vi "Update Channel Value.vi"(8 "error in (no error)":errorcluster, 9 "New Value":dbl, 10 "Channel Index":i32, 11 "Output Process in":refnum<class "Random Process.lvclass">) -> (0 "error out":errorcluster, 1 "# elements":u32, 2 "timed out?":bool, 3 "Output Process out":refnum<class "Random Process.lvclass">)   [LabVIEW 2019, in "TimingDRV Engine.lvlib" / "Random Process.lvclass"]
uses:
  Random Process.lvclass
  C:/Users/XEnderMD/Desktop/CD Project Tools/Source/Engine/Parent Classes/Process/Process.lvclass
  Random Process.lvclass/Random Process.ctl
  Parent Classes/Process/Process.lvclass/Process.ctl
  Parent Classes/Process/Process.lvclass
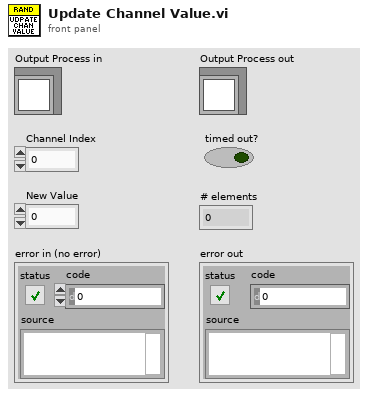
[diagram p1: front panel]
types:
  T1 = typedef "TimingDRV Engine.lvlib/Process.lvclass/Async Paramters.ctl" = cluster{"Device Reference":T2, "Device Clock":string, "Device Inputs FIFO":refnum<k33>, "Device Outputs FIFO":refnum<k33>, "CD Engine Event Ref":T3}
  T2 = typedef "Custom Device API.lvlib/Custom Device Item Ref.ctl" = u64
  T3 = typedef "Custom Device API.lvlib/Custom Device Engine Event Ref.ctl" = refnum<event-registration>
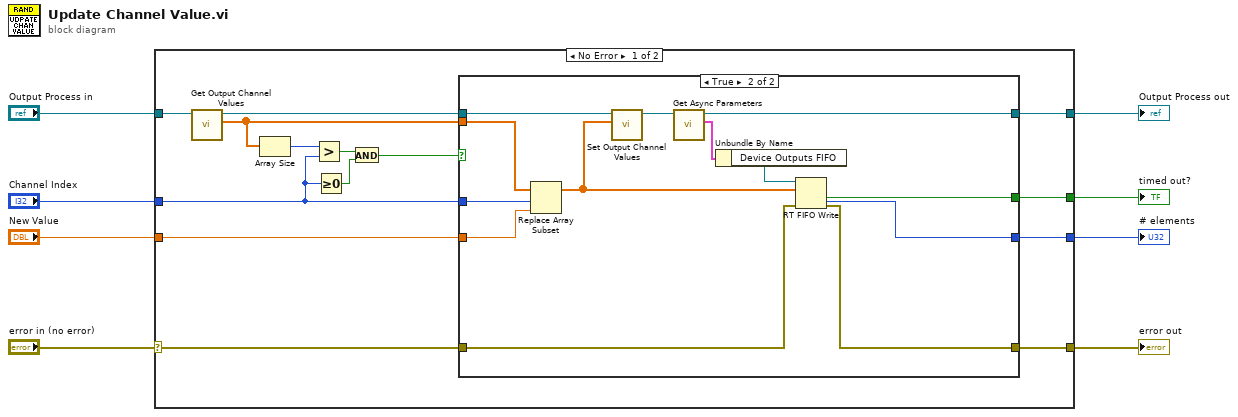
[diagram p0: block diagram]
diagram:
  n1 = case shown="No Error" "error in (no error)" {
    selector: "error in (no error)" -> [w15 w39]
    tunnel: [w22 w38] -> w8
    tunnel: [w21 _] -> w7
    tunnel: [w20 _] -> w6
    tunnel: [w19 w39] -> w5
    tunnel: "New Value" -> [w17 _]
    tunnel: "Channel Index" -> [w12 _]
    tunnel: "Output Process in" -> [w16 w38]
    frame No Error {
      n2 = call "Get Output Channel Values.vi"("Output Process in"=w16) -> ("Output Channel Values"=w14:dbl[], "Output Process out"=w18:refnum<class "Random Process.lvclass">)  [unwired: 9 in]
      n3 = Array Size(array=w14) -> (size(s)=w13:i32)
      n4 = Greater?(x=w13, y=w12) -> (0:w11:bool)
      n5 = Greater Or Equal To 0?(x=w12) -> (x >= 0?=w10:bool)
      n6 = And(x=w11, y=w10) -> (x .and. y?=w9:bool)
      n7 = case shown="True" w9 {
        tunnel: [w24 w27] -> w22
        tunnel: [_ w37] -> w21
        tunnel: [_ w36] -> w20
        tunnel: [w23 w29] -> w19
        tunnel: w18 -> [w24 w34]
        tunnel: w17 -> [_ w33]
        tunnel: w15 -> [w23 w32]
        tunnel: w14 -> [_ w31]
        tunnel: w12 -> [_ w30]
        frame False {
        }
        frame True {
          n8 = Replace Array Subset(array=w31, new element=w33, index=w30) -> (w35:dbl[])
          n9 = call "Set Output Channel Values.vi"("Output Channel Values"=w35, "Output Process in"=w34) -> ("Output Process out"=w28:refnum<class "Random Process.lvclass">)  [unwired: 9 in]
          n10 = call "Get Async Parameters.vi"("Process in"=w28) -> ("Async Parameters"=w26:T1, "Process out"=w27:refnum<class "Random Process.lvclass">)  [unwired: 9 in]
          n11 = Unbundle By Name(w26) -> ("Device Outputs FIFO"=w25:refnum<k33>)
          n12 = RT FIFO Write(0:w25, 1:w35, 3:w32) -> (7:w37:u32, 10:w36:bool, 11:w29:errorcluster)  [unwired: 2 in, 1 out]
        }
      }
    }
    frame Error {
    }
  }
  "Output Process out" <- w8
  "# elements" <- w7
  "timed out?" <- w6
  "error out" <- w5
